vi "Set_User_Limit.vi"(8 "error in":errorcluster, 10 "SetMin_Limit /Ohms":dbl=0.025, 11 "VISA name":refnum<visa-resource-name>="QR101") -> (0 "error out":errorcluster, 1 "valid":bool, 2 "output":T1, 3 "VISA out":refnum<visa-resource-name>)   [LabVIEW 2023, in "QR 10X Eastwood.lvlib"]
uses:
  <instrlib>/QR 10X Eastwood/QR 10X Eastwood.lvlib
panel:
  out "buffer":string
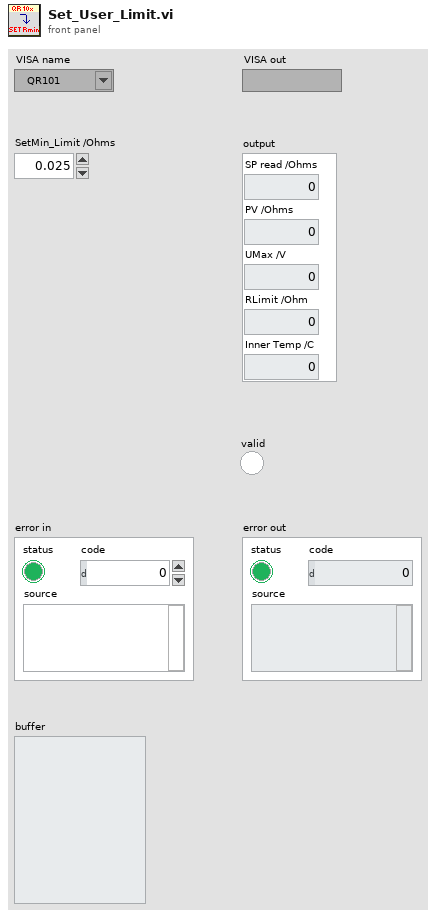
[diagram p1: front panel]
types:
  T1 = cluster{"SP read /Ohms":dbl, "PV /Ohms":dbl, "UMax /V":dbl, "RLimit /Ohm":dbl, "Inner Temp /C":dbl}
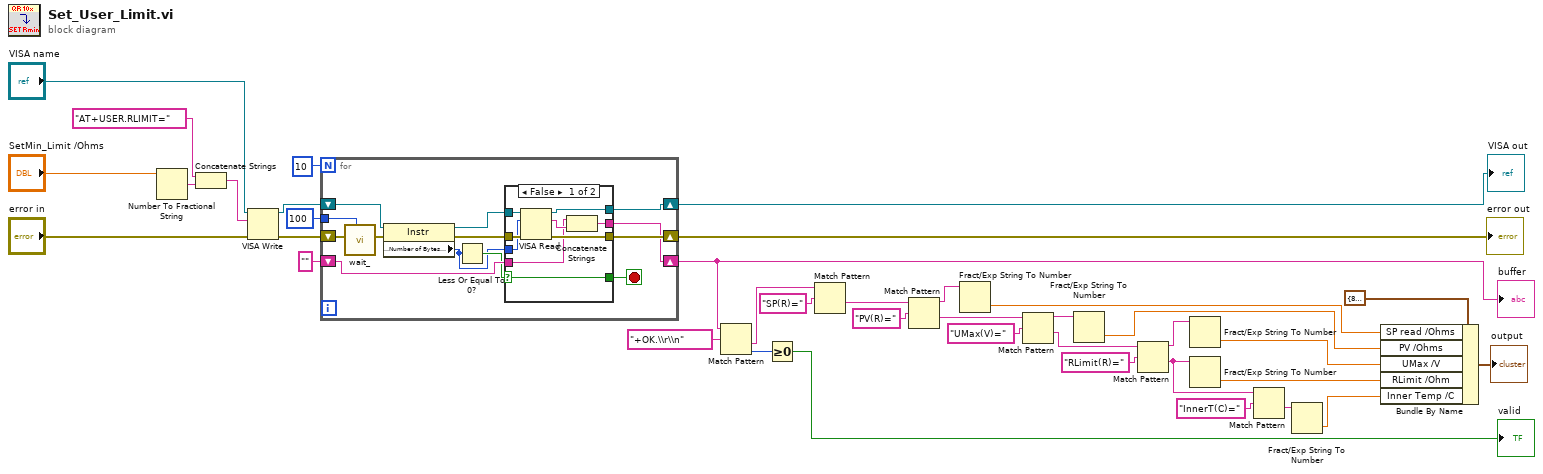
[diagram p0: block diagram]
diagram:
  n1 = Number To Fractional String(number="SetMin_Limit /Ohms") -> (F-format string=w17:string)  [unwired: 3 in]
  n2 = Concatenate Strings("AT+USER.RLIMIT=" ("write buffer"), w17) -> (w34:string)
  n3 = VISA Write(VISA resource name="VISA name", write buffer=w34, error in (no error)="error in") -> (VISA resource name out=w38:refnum<visa-resource-name>, error out=w33:errorcluster)  [unwired: 1 out]
  n4 = for {
    N: 10 -> [_]
    shift-right: [w47] -> w19
    shift-left: w38 -> [w51]
    shift-right: [w48] -> w18
    shift-left: w33 -> [w41]
    shift-right: [w46] -> w15
    shift-left: "" -> [w45]
    tunnel: u32 100 ("milliseconds to wait") -> [w39]
    stop <- w44 stop-if-true
    n5 = call "wait_.vi"("milliseconds to wait"=w39, "error in"=w41) -> ("error out"=w40:errorcluster)  [unwired: 9 in]
    n6 = property class="Instr"(reference=w51, error in=w40) -> (reference out=w49:refnum<visa-resource-name>, error out=w50:errorcluster, "Serial Settings:Number of Bytes at Serial Port"=w42:u32)
    n7 = Less Or Equal To 0?(x=w42) -> (x <= 0?=w43:bool)
    n8 = case shown="False" w43 {
      selector: w43 -> [w53 w61]
      tunnel: w50 -> [w60 w64]
      tunnel: w49 -> [w59 w63]
      tunnel: [w58 w64] -> w48
      tunnel: [w57 w63] -> w47
      tunnel: [w55 w62] -> w46
      tunnel: w45 -> [w54 w62]
      tunnel: [w53 w61] -> w44
      tunnel: w42 -> [w52 _]
      frame False {
        n9 = VISA Read(VISA resource name=w59, byte count=w52, error in (no error)=w60) -> (VISA resource name out=w57:refnum<visa-resource-name>, read buffer=w56:string, error out=w58:errorcluster)  [unwired: 1 out]
        n10 = Concatenate Strings(w54, w56) -> (w55:string)
      }
      frame True {
      }
    }
  }
  "buffer" <- w15
  "error out" <- w18
  "VISA out" <- w19
  n11 = Match Pattern(string=w15, regular expression="+OK.\\r\\n") -> (after substring=w23:string, offset past match=w14:i32)  [unwired: 1 in, 2 out]
  n12 = Greater Or Equal To 0?(x=w14) -> (x >= 0?=→"valid":bool)
  n13 = Match Pattern(string=w23, regular expression="SP(R)=") -> (after substring=w21:string)  [unwired: 1 in, 3 out]
  n14 = Match Pattern(string=w21, regular expression="PV(R)=") -> (before substring=w26:string, after substring=w29:string)  [unwired: 1 in, 2 out]
  n15 = Fract/Exp String To Number(string=w26) -> (number=w8:dbl)  [unwired: 3 in, 1 out]
  n16 = Match Pattern(string=w29, regular expression="UMax(V)=") -> (before substring=w25:string, after substring=w27:string)  [unwired: 1 in, 2 out]
  n17 = Fract/Exp String To Number(string=w25) -> (number=w7:dbl)  [unwired: 3 in, 1 out]
  n18 = Match Pattern(string=w27, regular expression="RLimit(R)=") -> (before substring=w24:string, after substring=w12:string)  [unwired: 1 in, 2 out]
  n19 = Fract/Exp String To Number(string=w24) -> (number=w6:dbl)  [unwired: 3 in, 1 out]
  n20 = Fract/Exp String To Number(string=w12) -> (number=w5:dbl)  [unwired: 3 in, 1 out]
  n21 = Match Pattern(string=w12, regular expression="InnerT(C)=") -> (after substring=w10:string)  [unwired: 1 in, 3 out]
  n22 = Fract/Exp String To Number(string=w10) -> (number=w4:dbl)  [unwired: 3 in, 1 out]
  n23 = Bundle By Name(cluster=T1 {"SP read /Ohms"=88.98, "PV /Ohms"=88.974, "UMax /V"=8.4, "RLimit /Ohm"=0.01, "Inner Temp /C"=0.01} ("Cluster"), "SP read /Ohms"=w8, "PV /Ohms"=w7, "UMax /V"=w6, "RLimit /Ohm"=w5, "Inner Temp /C"=w4) -> (→"output":T1)
